vi "Write Integer.vi"(7 "Section":string, 8 "error in":errorcluster, 9 "Value":i64, 10 "Key":string, 11 "config-base in":refnum<class "config-base.lvclass">) -> (0 "error out":errorcluster, 3 "config-base out":refnum<class "config-base.lvclass">)   [LabVIEW 2022 SP3, in "hse-config.lvlib" / "config-base.lvclass"]
doc: "Set a integer config key.\n\n____\nHAMPEL SOFTWARE ENGINEERING v3.8.0 (2023-12-18 14:41)"
uses:
  config-base.lvclass
  config-base.lvclass/config-base.ctl
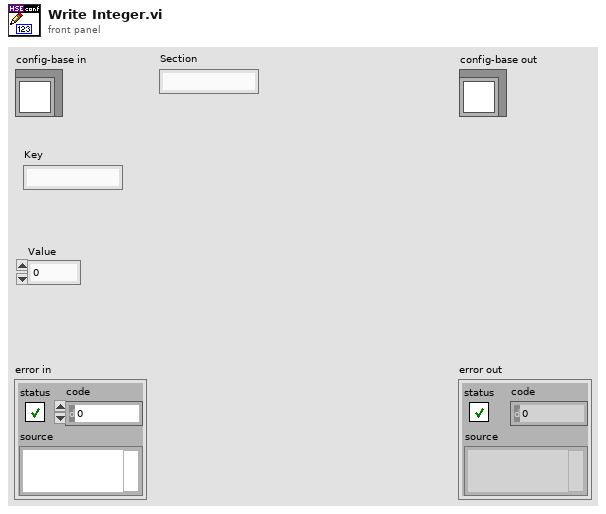
[diagram p1: front panel]
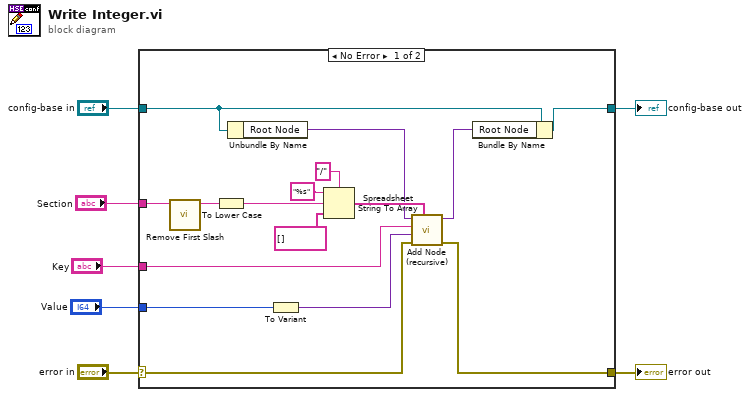
[diagram p0: block diagram]
diagram:
  n1 = case shown="No Error" "error in" {
    selector: "error in" -> [w15 w25]
    tunnel: [w14 w25] -> w6
    tunnel: [w12 w24] -> w4
    tunnel: "config-base in" -> [w13 w24]
    tunnel: "Section" -> [w10 _]
    tunnel: "Key" -> [w18 _]
    tunnel: "Value" -> [w17 _]
    frame No Error {
      n2 = call "Remove First Slash.vi"("Section"=w10) -> ("result string"=w9:string)  [unwired: 10 in]
      n3 = To Lower Case(string=w9) -> (all lower case string=w8:string)
      n4 = Unbundle By Name(w13) -> ("Root Node"=w19:variant)
      n5 = To Variant(anything=w17) -> (Variant=w16:variant)
      n6 = Spreadsheet String To Array(delimiter (Tab)="/" ("Split Pattern"), format string="%s", spreadsheet string=w8, array type (2D Dbl)=string[] []) -> (array=w23:string[])
      n7 = call "Add Node (recursive).vi"("Section"=w23, "error in"=w15, "Value"=w16, "Key"=w18, "Node in"=w19) -> ("error out"=w14:errorcluster, "Node out"=w11:variant)  [unwired: 5 in]
      n8 = Bundle By Name(cluster=w13, "Root Node"=w11) -> (w12:refnum<class "config-base.lvclass">)
    }
    frame Error {
    }
  }
  "error out" <- w6
  "config-base out" <- w4
